vi "Path Index.vi"(11 "JSON Path":string) -> (3 "Index":i32)   [LabVIEW 2019, in "labview_json.lvlib"]
uses:
  labview_json.lvlib
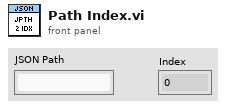
[diagram p1: front panel]
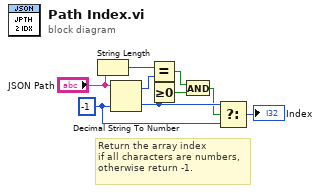
[diagram p0: block diagram]
diagram:
  w5 = -1 ("default (0 I32)")
  # "Return the array index\nif all characters are numbers,\notherwise return -1."
  n1 = String Length(string="JSON Path") -> (length=w8:i32)
  n2 = Decimal String To Number(string="JSON Path", default (0L)=w5) -> (offset past number=w7:i32, number=w3:i32)  [unwired: 1 in]
  n3 = Equal?(x=w8, y=w7) -> (x = y?=w6:bool)
  n4 = Greater Or Equal To 0?(x=w3) -> (x >= 0?=w1:bool)
  n5 = And(x=w6, y=w1) -> (x .and. y?=w2:bool)
  n6 = Select(t=w3, s=w2, f=w5) -> (s? t:f=→"Index":i32)
